vi "ClearCompileCache--function.vi"(8 "error in":errorcluster, 11 "-Cache":T1) -> (0 "error out":errorcluster)   [LabVIEW 2020, in "CICD.lvlib"]
doc: "Clear the compiled object cache with a flag to specify which cache to clear user/application/both (default is clear all compiled object cache)."
uses:
  CICD.lvlib
  Cache--enum.ctl
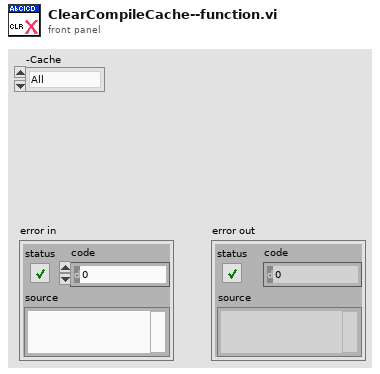
[diagram p1: front panel]
types:
  T1 = typedef "CICD.lvlib/Cache--enum.ctl" = enum16{"All", "User", "AppBuilder"}
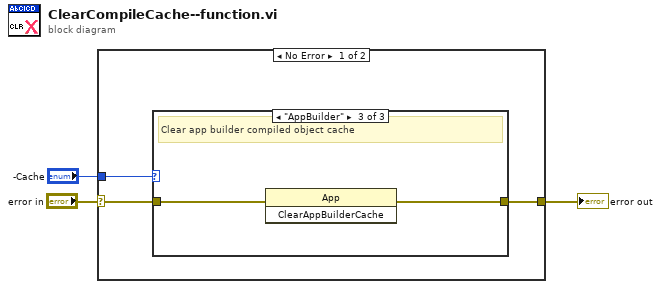
[diagram p0: block diagram]
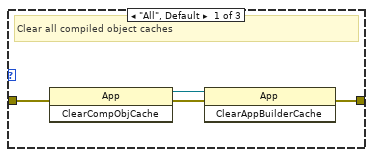
[diagram p2: hidden frame]
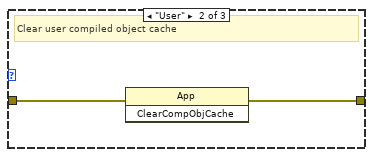
[diagram p3: hidden frame]
diagram:
  n1 = case shown="No Error" "error in" {
    selector: "error in" -> [w4 w15]
    tunnel: [w6 w15] -> w3
    tunnel: "-Cache" -> [w5 _]
    frame No Error {
      n2 = case shown="\"AppBuilder\"" w5 {
        tunnel: w4 -> [w10 w12 w14]
        tunnel: [w8 w11 w13] -> w6
        frame "All", Default {
          # "Clear all compiled object caches"
          n3 = invoke class="App" method="ClearCompObjCache"(error in=w10) -> (reference out=w7:refnum<vi>, error out=w9:errorcluster)  [unwired: 2 in, 1 out]
          n4 = invoke class="App" method="ClearAppBuilderCache"(reference=w7, error in=w9) -> (error out=w8:errorcluster)  [unwired: 1 in, 2 out]
        }
        frame "User" {
          # "Clear user compiled object cache"
          n5 = invoke class="App" method="ClearCompObjCache"(error in=w12) -> (error out=w11:errorcluster)  [unwired: 2 in, 2 out]
        }
        frame "AppBuilder" {
          # "Clear app builder compiled object cache"
          n6 = invoke class="App" method="ClearAppBuilderCache"(error in=w14) -> (error out=w13:errorcluster)  [unwired: 2 in, 2 out]
        }
      }
    }
    frame Error {
    }
  }
  "error out" <- w3
